vi "APS relative arc move 3pe.vi"(0 "Dimension":i32, 1 "Max_Arc_Speed":i32, 5 "Axis_ID_Array":i32, 7 "Pass_PosOffset_Array":i32, 9 "End_PosOffset_Array":i32, 11 "error in (no error)":errorcluster caption="错误输入（无错误）") -> (4 "function return":i32, 6 "Axis_ID_Array out":i32, 8 "Pass_PosOffset_Array out":i32, 10 "End_PosOffset_Array out":i32, 15 "error out":errorcluster caption="错误输出")   [LabVIEW 2011, in "APS168.lvlib"]
doc: "I32 FNTYPE APS_relative_arc_move_3pe(I32 Dimension, I32 *Axis_ID_Array, I32 *Pass_PosOffset_Array, I32 *End_PosOffset_Array, I32 Max_Arc_Speed );"
uses:
  APS168.lvlib
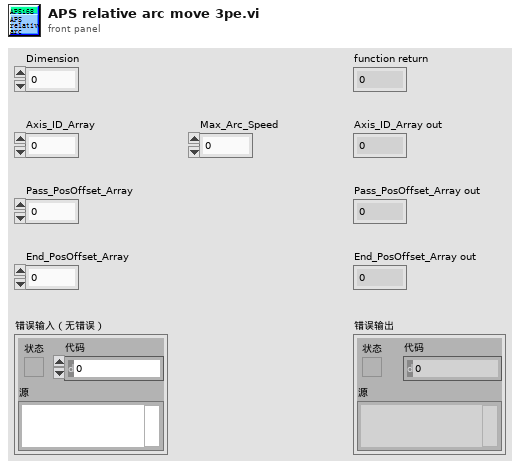
[diagram p1: front panel]
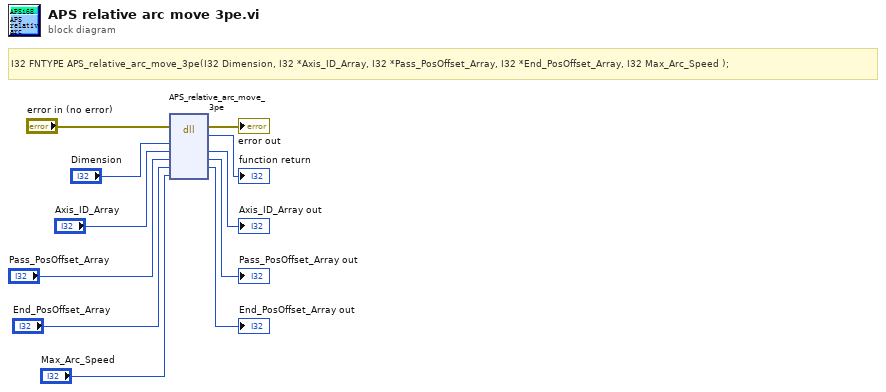
[diagram p0: block diagram]
diagram:
  # "I32 FNTYPE APS_relative_arc_move_3pe(I32 Dimension, I32 *Axis_ID_Array, I32 *Pass_PosOffset_Array, I32 *End_PosOffset_Array, I32 Max_Arc_Speed );"
  n1 = dll-call lib="PTH1Labs E软件ADLINK 204CAPS_1_7_1_LIB line 连续运动204APS168.*" fn="APS_relative_arc_move_3pe"(error in="error in (no error)", "Dimension"="Dimension", "Axis_ID_Array"="Axis_ID_Array", "Pass_PosOffset_Array"="Pass_PosOffset_Array", "End_PosOffset_Array"="End_PosOffset_Array", "Max_Arc_Speed"="Max_Arc_Speed") -> (error out=→"error out":errorcluster, →"function return":i32, "Axis_ID_Array"=→"Axis_ID_Array out":i32, "Pass_PosOffset_Array"=→"Pass_PosOffset_Array out":i32, "End_PosOffset_Array"=→"End_PosOffset_Array out":i32)  [unwired: 4 in, 1 out]
